vi "SMO.Template.TestLauncher.vi"() -> ()   [LabVIEW 2013, in "SMO.Template.lvclass"]
uses:
  SMO.Template.lvclass
  SMO/SMO.lvclass
panel:
  out "error out":errorcluster
  in  "Stop":bool
  # "SMO Test Launcher"
  # "For instructions on how to use the JKI State Machine Objects, examples and video tutorials, visit:\nhttp://jki.net/state-machine-objects/\n\nJKI State Machine Objects™\nhttp://jki.net/state-machine-objects/\nCopyright (C) 2005-2015, JKI <info@jki.net>\nALL RIGHTS RESERVED"
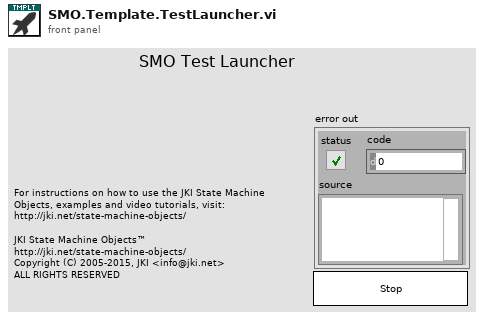
[diagram p1: front panel]
types:
  T1 = cluster{"SMO.Template Public Events":refnum<event-registration>}
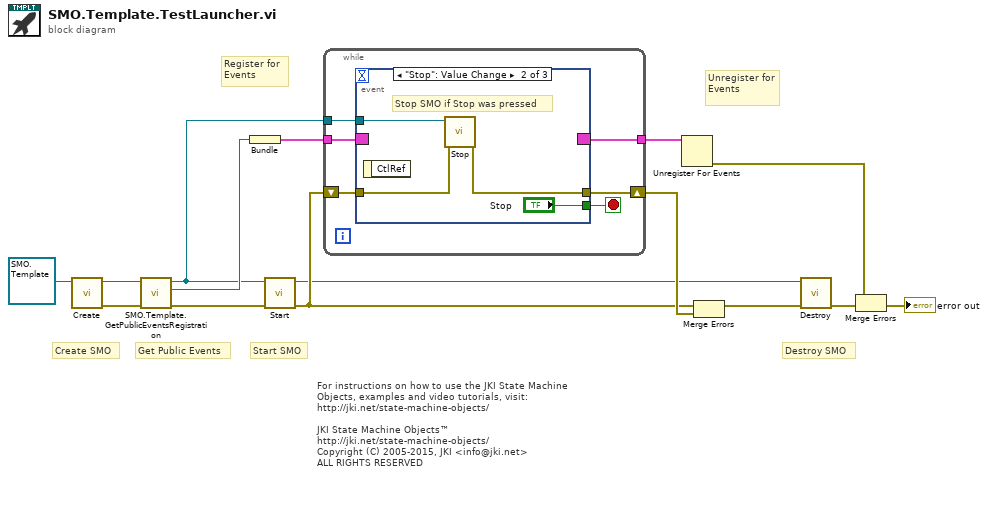
[diagram p0: block diagram]
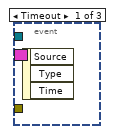
[diagram p2: hidden frame]
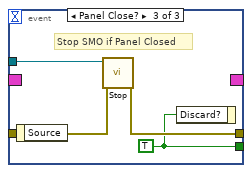
[diagram p3: hidden frame]
diagram:
  # "For instructions on how to use the JKI State Machine Objects, examples and video tutorials, visit:\nhttp://jki.net/state-machine-objects/\n\nJKI State Machine Objects™\nhttp://jki.net/state-machine-objects/\nCopyright (C) 2005-2015, JKI <info@jki.net>\nALL RIGHTS RESERVED"
  # "Get Public Events"
  # "Start SMO"
  # "Destroy SMO"
  # "Create SMO"
  # "Unregister for Events"
  # "Register for Events"
  n1 = call "Create.vi"("SMO"=refnum<class "SMO.Template.lvclass"> refnum ("SMO.Template.lvclass")) -> ("error out"=w7:errorcluster, "SMO out"=w8:refnum<class "SMO.Template.lvclass">)  [unwired: 9 in]
  n2 = call "SMO.Template.GetPublicEventsRegistration.vi"("error in (no error)"=w7, "SMO"=w8) -> ("error out"=w6:errorcluster, "SMO.Template Public Events"=w5:refnum<event-registration>, "SMO out"=w1:refnum<class "SMO.Template.lvclass">)  [unwired: 7 in]
  n3 = Bundle("SMO.Template Public Events"=w5) -> (w14:T1)  [unwired: 1 in]
  n4 = call "Start.vi"("error in (no error)"=w6, "SMO"=w1) -> ("error out"=w4:errorcluster, "SMO out"=w3:refnum<class "SMO.Template.lvclass">)  [unwired: 8 in]
  n5 = while {
    shift-right: [w20] -> w13
    shift-left: w4 -> [w19]
    tunnel: w14 -> [w18]
    tunnel: [w17] -> w15
    tunnel: w1 -> [w16]
    stop <- w21 stop-if-true
    n6 = event shown="[1] \"Stop\": Value Change" {
      selector: w18 -> [_ _ _]
      dyn-events: [_ _ _] -> w17
      timeout: _ -> [_ _ _]
      tunnel: [_ "Stop" w26] -> w21
      tunnel: w16 -> [_ w24 w29]
      tunnel: [_ w23 w28] -> w20
      tunnel: w19 -> [_ w22 w27]
      event Timeout {
        n7 = event-data() -> ()  [unwired: 1 in, 3 out]
      }
      event "Stop": Value Change {
        # "Stop SMO if Stop was pressed"
        n8 = event-data() -> ()  [unwired: 1 in, 1 out]
        n9 = call "Stop.vi"("error in (no error)"=w22, "SMO"=w24) -> ("error out"=w23:errorcluster)  [unwired: 8 in, 1 out]
      }
      event Panel Close? {
        w26 = TRUE ("OK")
        # "Stop SMO if Panel Closed"
        n10 = event-data() -> ()  [unwired: 1 in, 1 out]
        n11 = call "Stop.vi"("error in (no error)"=w27, "SMO"=w29) -> ("error out"=w28:errorcluster)  [unwired: 8 in, 1 out]
        n12 = event-data("Discard?"=w26) -> ()  [unwired: 1 in, 1 out]
      }
    }
  }
  n13 = Unregister For Events(event registration refnum=w15) -> (error out=w12:errorcluster)  [unwired: 1 in]
  n14 = Merge Errors(w4, w13) -> (w2:errorcluster)
  n15 = call "Destroy.vi"("error in (no error)"=w2, "SMO"=w3) -> ("error out"=w10:errorcluster)  [unwired: 9 in]
  n16 = Merge Errors(w12, w10) -> (→"error out":errorcluster)
